vi "Discover_Switch.vi"(8 "error in":errorcluster {"code" format="%.0x"}, 11 "Session In":refnum<visa-resource-name>="TCPIP0::10.0.1.24::inst0::INSTR") -> (0 "error out":errorcluster, 2 "Success?(t)":bool, 3 "Session Out":refnum<visa-resource-name>)   [LabVIEW 2018]
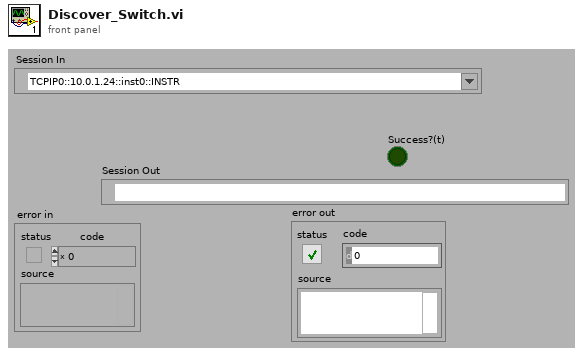
[diagram p1: front panel]
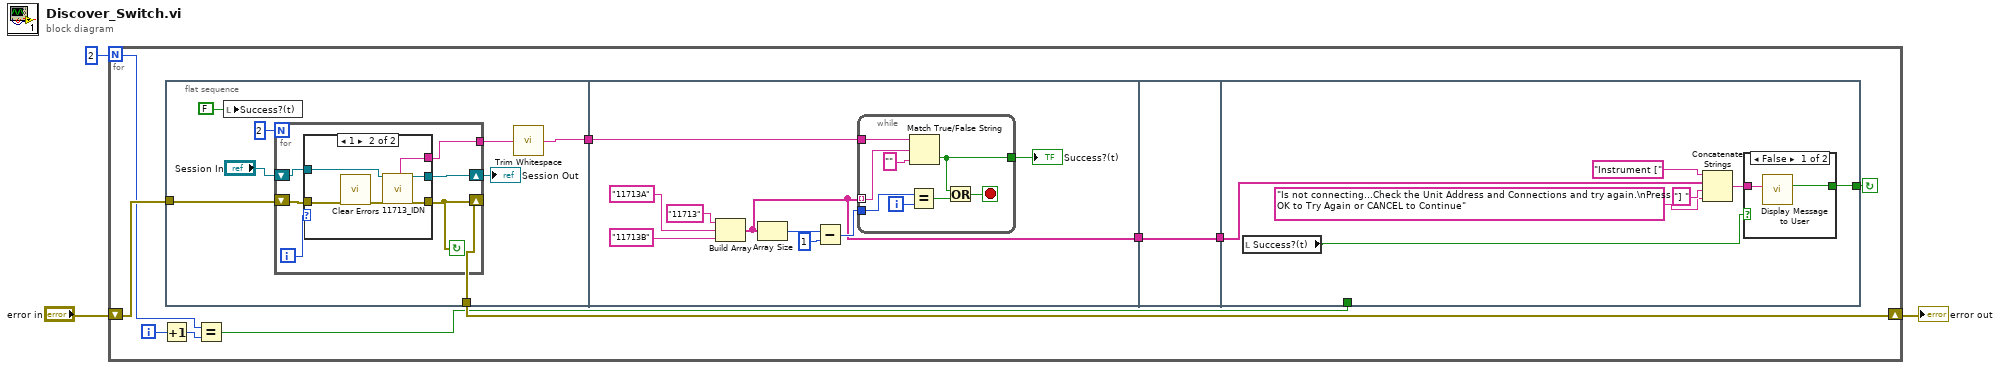
[diagram p0: block diagram]
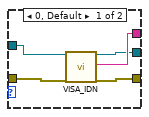
[diagram p2: hidden frame]
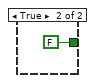
[diagram p3: hidden frame]
diagram:
  n1 = for {
    N: 2 -> [w6]
    shift-right: [w8] -> w1
    shift-left: "error in" -> [w9]
    i -> [w7]
    stop <- w12 continue-if-true
    n2 = Increment(x=w7) -> (x+1=w5:i32)
    n3 = flat-sequence {
      tunnel: [w19] -> w13
      tunnel: w9 -> [w17]
      tunnel: [w16] -> w8
      tunnel: w13 -> [w44]
      tunnel: [w43] -> w11
      tunnel: w11 -> [w56]
      tunnel: [w56] -> w10
      tunnel: w10 -> [w62]
      tunnel: [w58] -> w12
      tunnel: w4 -> [_]
      frame #0 {
        n4 = local write "Success?(t)"(FALSE ("Success?(t)")) -> ()
        n5 = for {
          N: 2 -> [_]
          tunnel: [w27] -> w21
          shift-right: [w25] -> w18
          shift-left: "Session In" -> [w26]
          shift-right: [w22] -> w16
          shift-left: w17 -> [w24]
          i -> [w23]
          stop <- w22 continue-if-true
          n6 = case shown="1" w23 {
            tunnel: [w32 w36] -> w27
            tunnel: w26 -> [w31 w37]
            tunnel: [w30 w38] -> w25
            tunnel: [w29 w35] -> w22
            tunnel: w24 -> [w28 w33]
            frame 0, Default {
              n7 = call "VISA_IDN.vi"("Session In"=w31, "error in"=w28) -> ("Session Out"=w30:refnum<visa-resource-name>, "Model"=w32:string, "error out"=w29:errorcluster)  [unwired: 11 in, 4 out]
            }
            frame 1 {
              n8 = call <vilib>:"Clear Errors.vi"("error in (no error)"=w33) -> ("error out"=w34:errorcluster)  [unwired: 5 in, 1 out]
              n9 = call "11713_IDN.vi"("Session In"=w37, "error in"=w34) -> ("model out(str)"=w36:string, "Session Out"=w38:refnum<visa-resource-name>, "error out"=w35:errorcluster)  [unwired: 14 in, 1 out]
            }
          }
        }
        "Session Out" <- w18
        n10 = call <vilib>:"Trim Whitespace.vi"("string"=w21) -> ("trimmed string"=w19:string)  [unwired: 1 in]
      }
      frame #1 {
        n11 = Build Array("11713" ("element"), "11713A" ("element"), "11713B" ("true string")) -> (w43:string[])
        n12 = Array Size(array=w43) -> (size(s)=w47:i32)
        n13 = Subtract(x=w47, y=1) -> (x-y=w45:i32)
        n14 = while {
          tunnel: w43 -> [w54] mode=indexing
          tunnel: w44 -> [w53]
          tunnel: [w52] -> w39
          tunnel: w45 -> [w48]
          i -> [w49]
          stop <- w51 stop-if-true
          n15 = Equal?(x=w48, y=w49) -> (x = y?=w50:bool)
          n16 = Match True/False String(2:"" ("false string"), 3:w54, 4:w53) -> (0:w52:bool)  [unwired: 1 out]
          n17 = Or(x=w52, y=w50) -> (x .or. y?=w51:bool)
        }
        "Success?(t)" <- w39
      }
      frame #2 {
      }
      frame #3 {
        n18 = local read "Success?(t)"() -> (w57:bool)
        n19 = Concatenate Strings("Instrument [" ("string"), w62, "] " ("string"), "Is not connecting...Check the Unit Address and Connections and try again.\nPress OK to Try Again or CANCEL to Continue" ("string")) -> (w59:string)
        n20 = case shown="False" w57 {
          tunnel: w59 -> [w65 _]
          tunnel: [w64 FALSE ("OK")] -> w58
          frame False {
            n21 = call "Display Message to User"("Message"=w65) -> ("OK"=w64:bool)  [unwired: 9 in, 1 out]
          }
          frame True {
          }
        }
      }
    }
    n22 = Equal?(x=w6, y=w5) -> (x = y?=w4:bool)
  }
  "error out" <- w1
